vi "Parse LVClasses by Type.vi"(11 "Input":string) -> (3 "Relative Paths":path[](array[path]))   [LabVIEW 2020, in "Test Method Finding Test.lvclass"]
uses:
  Test Method Finding Test.lvclass
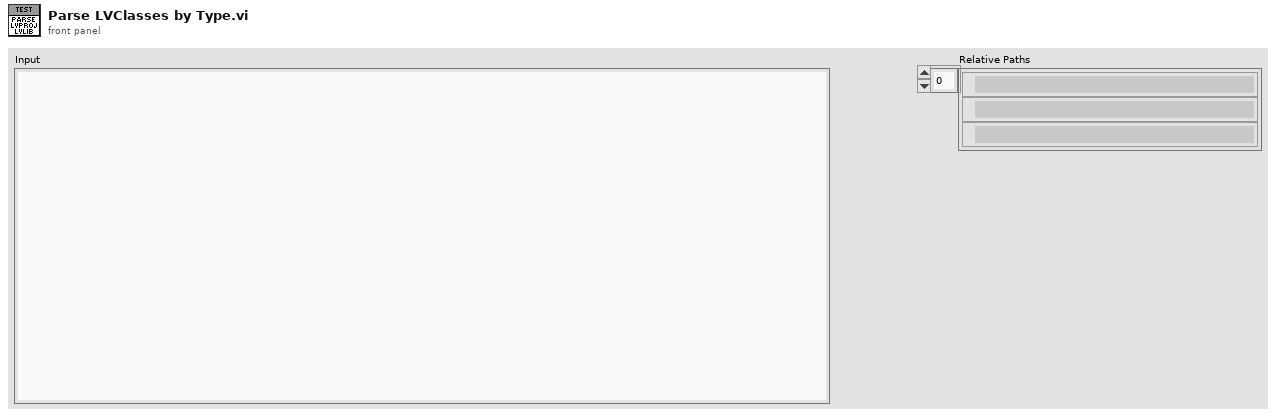
[diagram p1: front panel]
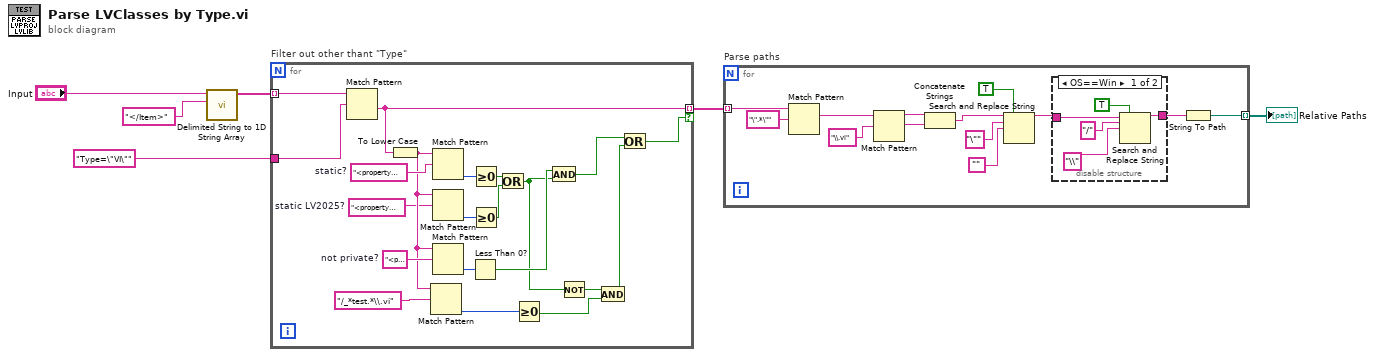
[diagram p0: block diagram]
diagram:
  n1 = call <vilib>:"Delimited String to 1D String Array.vi"("delimiter"="</Item>" ("regular expression"), "delimited string"="Input") -> ("string array"=w5:string[])  [unwired: 9 in]
  n2 = for "Filter out other thant \"Type\"" {
    tunnel: w5 -> [w27] mode=indexing
    tunnel: [w22] -> w2 mode=indexing if=w14
    tunnel: "Type=\"VI\"" ("regular expression") -> [w26]
    w9 = "<property name=\"ni.classitem.invokeusage\" type=\"uint\">0"  # static LV2025?
    w21 = "<property name=\"ni.classitem.methodscope\" type=\"uint\">2"  # not private?
    w25 = "<property name=\"ni.classitem.isstaticmethod\" type=\"bool\">true"  # static?
    n3 = Match Pattern(string=w27, regular expression=w26) -> (after substring=w22:string)  [unwired: 1 in, 3 out]
    n4 = To Lower Case(string=w22) -> (all lower case string=w10:string)
    n5 = Match Pattern(string=w10, regular expression="/_*test.*\\.vi") -> (offset past match=w18:i32)  [unwired: 1 in, 3 out]
    n6 = Match Pattern(string=w10, regular expression=w25) -> (offset past match=w24:i32)  [unwired: 1 in, 3 out]
    n7 = Match Pattern(string=w10, regular expression=w9) -> (offset past match=w11:i32)  [unwired: 1 in, 3 out]
    n8 = Match Pattern(string=w10, regular expression=w21) -> (offset past match=w23:i32)  [unwired: 1 in, 3 out]
    n9 = Less Than 0?(x=w23) -> (x < 0?=w20:bool)
    n10 = Greater Or Equal To 0?(x=w24) -> (x >= 0?=w17:bool)
    n11 = Greater Or Equal To 0?(x=w11) -> (x >= 0?=w7:bool)
    n12 = Or(x=w17, y=w7) -> (x .or. y?=w8:bool)
    n13 = Greater Or Equal To 0?(x=w18) -> (x >= 0?=w15:bool)
    n14 = And(x=w20, y=w8) -> (x .and. y?=w13:bool)
    n15 = Not(x=w8) -> (.not. x?=w16:bool)
    n16 = And(x=w16, y=w15) -> (x .and. y?=w12:bool)
    n17 = Or(x=w13, y=w12) -> (x .or. y?=w14:bool)
  }
  n18 = for "Parse paths" {
    tunnel: w2 -> [w40] mode=indexing
    tunnel: [w35] -> w3 mode=indexing
    n19 = Match Pattern(string=w40, regular expression="\".*\"") -> (match substring=w29:string)  [unwired: 1 in, 3 out]
    n20 = Match Pattern(string=w29, regular expression="\\.vi") -> (before substring=w31:string, match substring=w30:string)  [unwired: 1 in, 2 out]
    n21 = Concatenate Strings(w31, w30) -> (w28:string)
    n22 = Search and Replace String(replace all?=TRUE ("replace all? (F)"), input string=w28, search string="\"", replace string="") -> (result string=w34:string)  [unwired: 4 in, 3 out]
    n23 = disable-structure shown="OS==Win" {
      disable-tunnel: [w44 w46] -> w33
      disable-tunnel: w34 -> [w43 w46]
      frame condition #0 (active) {
        n24 = Search and Replace String(replace all?=TRUE ("replace all? (F)"), input string=w43, search string="/", replace string="\\" ("search string")) -> (result string=w44:string)  [unwired: 4 in, 3 out]
      }
      frame condition #1 {
      }
    }
    n25 = String To Path(string=w33) -> (path=w35:path)
  }
  "Relative Paths" <- w3
